vi "COMI Digit14To Volt.vi"(9 "vmax":sgl, 10 "vmin":sgl, 11 "digit":i16) -> (3 "function return":sgl)   [LabVIEW 2017, in "Comidll.lvlib"]
doc: "float (COMI_Digit14ToVolt) (short digit, float vmin, float vmax);"
uses:
  <userlib>/Comidll/Comidll.lvlib
  <userlib>/Comidll/Comidll.dll
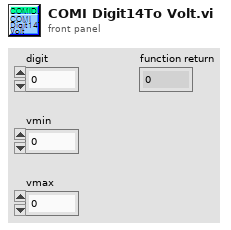
[diagram p1: front panel]
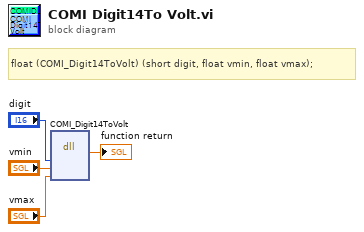
[diagram p0: block diagram]
diagram:
  # "float\t(COMI_Digit14ToVolt) (short digit, float vmin, float vmax);"
  n1 = dll-call lib="C:/Program Files/National Instruments/LabVIEW 2017/user.lib/Comidll/Comidll.*" fn="COMI_Digit14ToVolt"("digit"="digit", "vmin"="vmin", "vmax"="vmax") -> (→"function return":sgl)  [unwired: 6 in, 2 out]
